vi "Write Flange 1 Depth.vi"(8 "error in (no error)":errorcluster, 10 "Flange1Depth":u32, 11 "MultiSegmentPipe.lvclass in":refnum<class "MultiSegmentPipe.lvclass">) -> (0 "error out":errorcluster, 3 "MultiSegmentPipe.lvclass out":refnum<class "MultiSegmentPipe.lvclass">)   [LabVIEW 2015, in "MultiSegmentPipe.lvclass"]
uses:
  MultiSegmentPipe.lvclass
  MultiSegmentPipe.lvclass/MultiSegmentPipe.ctl
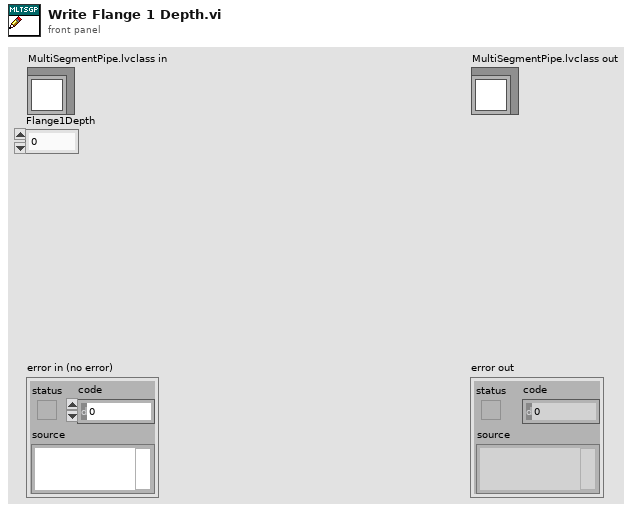
[diagram p1: front panel]
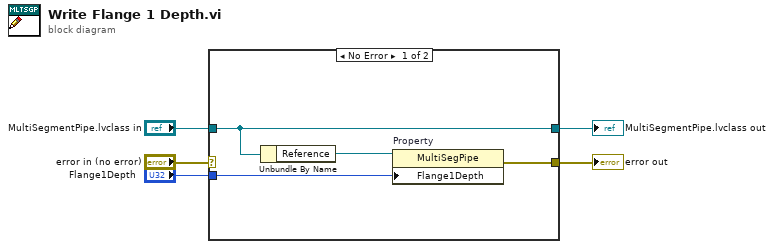
[diagram p0: block diagram]
diagram:
  n1 = case shown="No Error" "error in (no error)" {
    selector: "error in (no error)" -> [_ w11]
    tunnel: [w9 w11] -> w4
    tunnel: [w7 w10] -> w2
    tunnel: "MultiSegmentPipe.lvclass in" -> [w7 w10]
    tunnel: "Flange1Depth" -> [w8 _]
    frame No Error {
      n2 = Unbundle By Name(w7) -> ("Reference"=w6:refnum<vi>)
      n3 = property on="Property" class="MultiSegPipe"(reference=w6, "Flange1Depth"=w8) -> (error out=w9:errorcluster)  [unwired: 1 in, 1 out]
    }
    frame Error {
    }
  }
  "error out" <- w4
  "MultiSegmentPipe.lvclass out" <- w2
